vi "Get Value.vi"(8 "error in (no error)":errorcluster, 11 "DA Child A in":refnum<class "DA Child A.lvclass">) -> (0 "error out":errorcluster, 2 "Value":string, 3 "DA Child A out":refnum<class "DA Child A.lvclass">)   [LabVIEW 2020, in "Display As.lvlib" / "DA Child A.lvclass"]
uses:
  DA Child A.lvclass
  DA Child A.lvclass/DA Child A.ctl
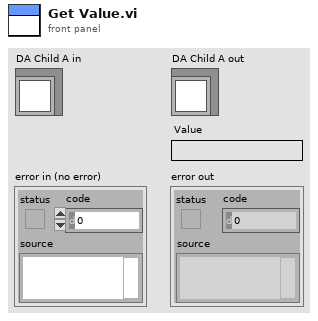
[diagram p1: front panel]
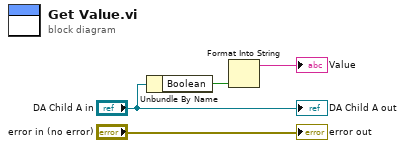
[diagram p0: block diagram]
diagram:
  n1 = Unbundle By Name("DA Child A in") -> ("Boolean"=w2:bool)
  n2 = Format Into String(w2) -> (resulting string=→"Value":string)  [unwired: 3 in, 1 out]
  "error out" <- "error in (no error)"
  "DA Child A out" <- "DA Child A in"
